vi "Impedance tube v1.0.2.vi"() -> ()   [LabVIEW 2021]
uses:
  <vilib>/Analysis/1siggen.llb/Ramp Pattern by Samples.vi
  <vilib>/express/express analysis/Spectral/Block/exnSpectralBlock spectral measurements RMS poly.vi
  <vilib>/express/express analysis/Spectral/Block/exnSpectralBlock spectral measurements RMS WFM.vi
  <vilib>/express/express analysis/Spectral/Block/exnSpectralBlock spectral measurements RMS DDT.vi
  <vilib>/Utility/file.llb/Write Delimited Spreadsheet (DBL).vi
  <vilib>/express/express arith-compare/Formula/XNode/ExpressFormulaBlockNode.xnode
  <vilib>/express/express analysis/Spectral/XNode/ExpressSpectralMeasurementsBlockNode.xnode
  <vilib>/Analysis/NI_AALPro.lvlib
  <vilib>/Analysis/NI_AALBase.lvlib
  <vilib>/measure/NI_MABase.lvlib
panel:
  out "Dout":cluster{"f0":dbl, "df":dbl, "magnitude":dbl[]}(graph)
  out "Probe":dbl[](graph)
  out "Rr":dbl[](graph)
  out "Absorption coeff":dbl[](graph)
  in  "number of samples":i32=2048
  out "MIC 2":dynamicdata(graph)
  out "MIC 2":dbl
  out "FFT1":dynamicdata(graph)
  out "MIC 1":dynamicdata(graph)
  out "MIC 1":dbl
  in  "stop (F)":bool
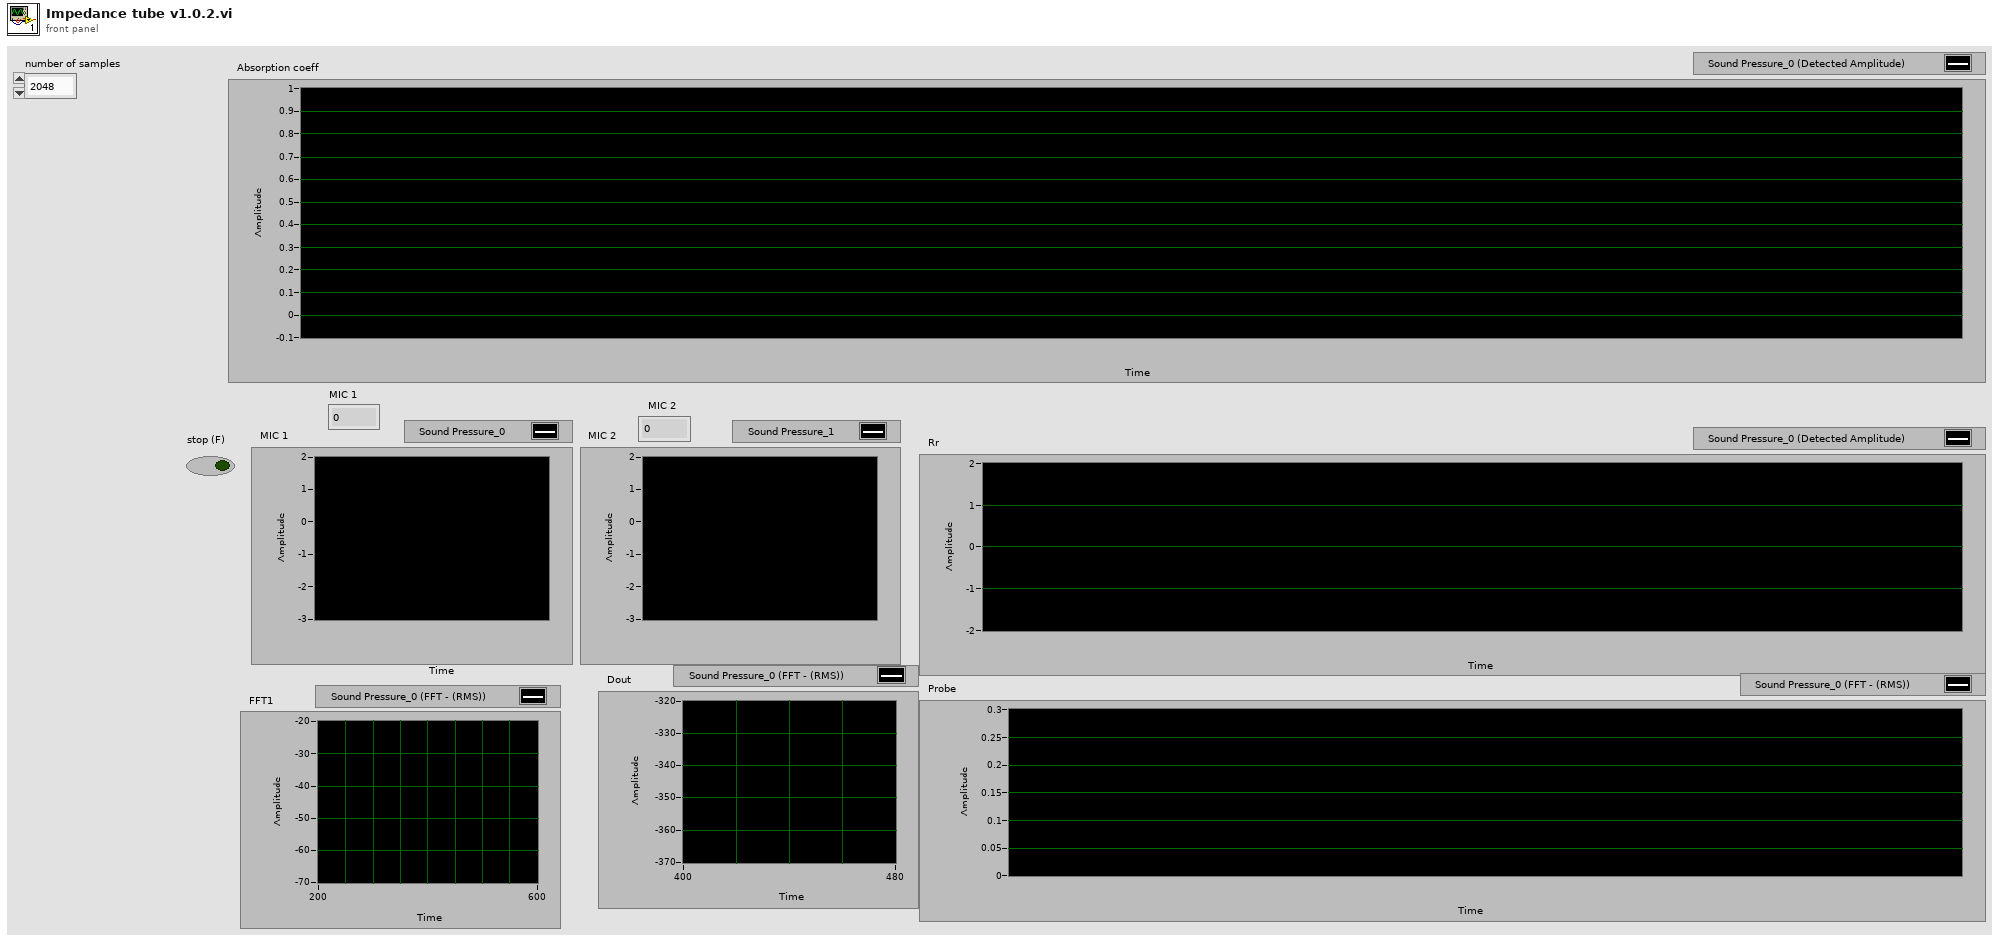
[diagram p1: front panel]
types:
  T1 = cluster{"averaging mode":u16, "weighting mode":u16, "number of averages":u32}
  T2 = cluster{"dB On (F)":bool, "unwrap phase (F)":bool, "convert to degree (F)":bool}
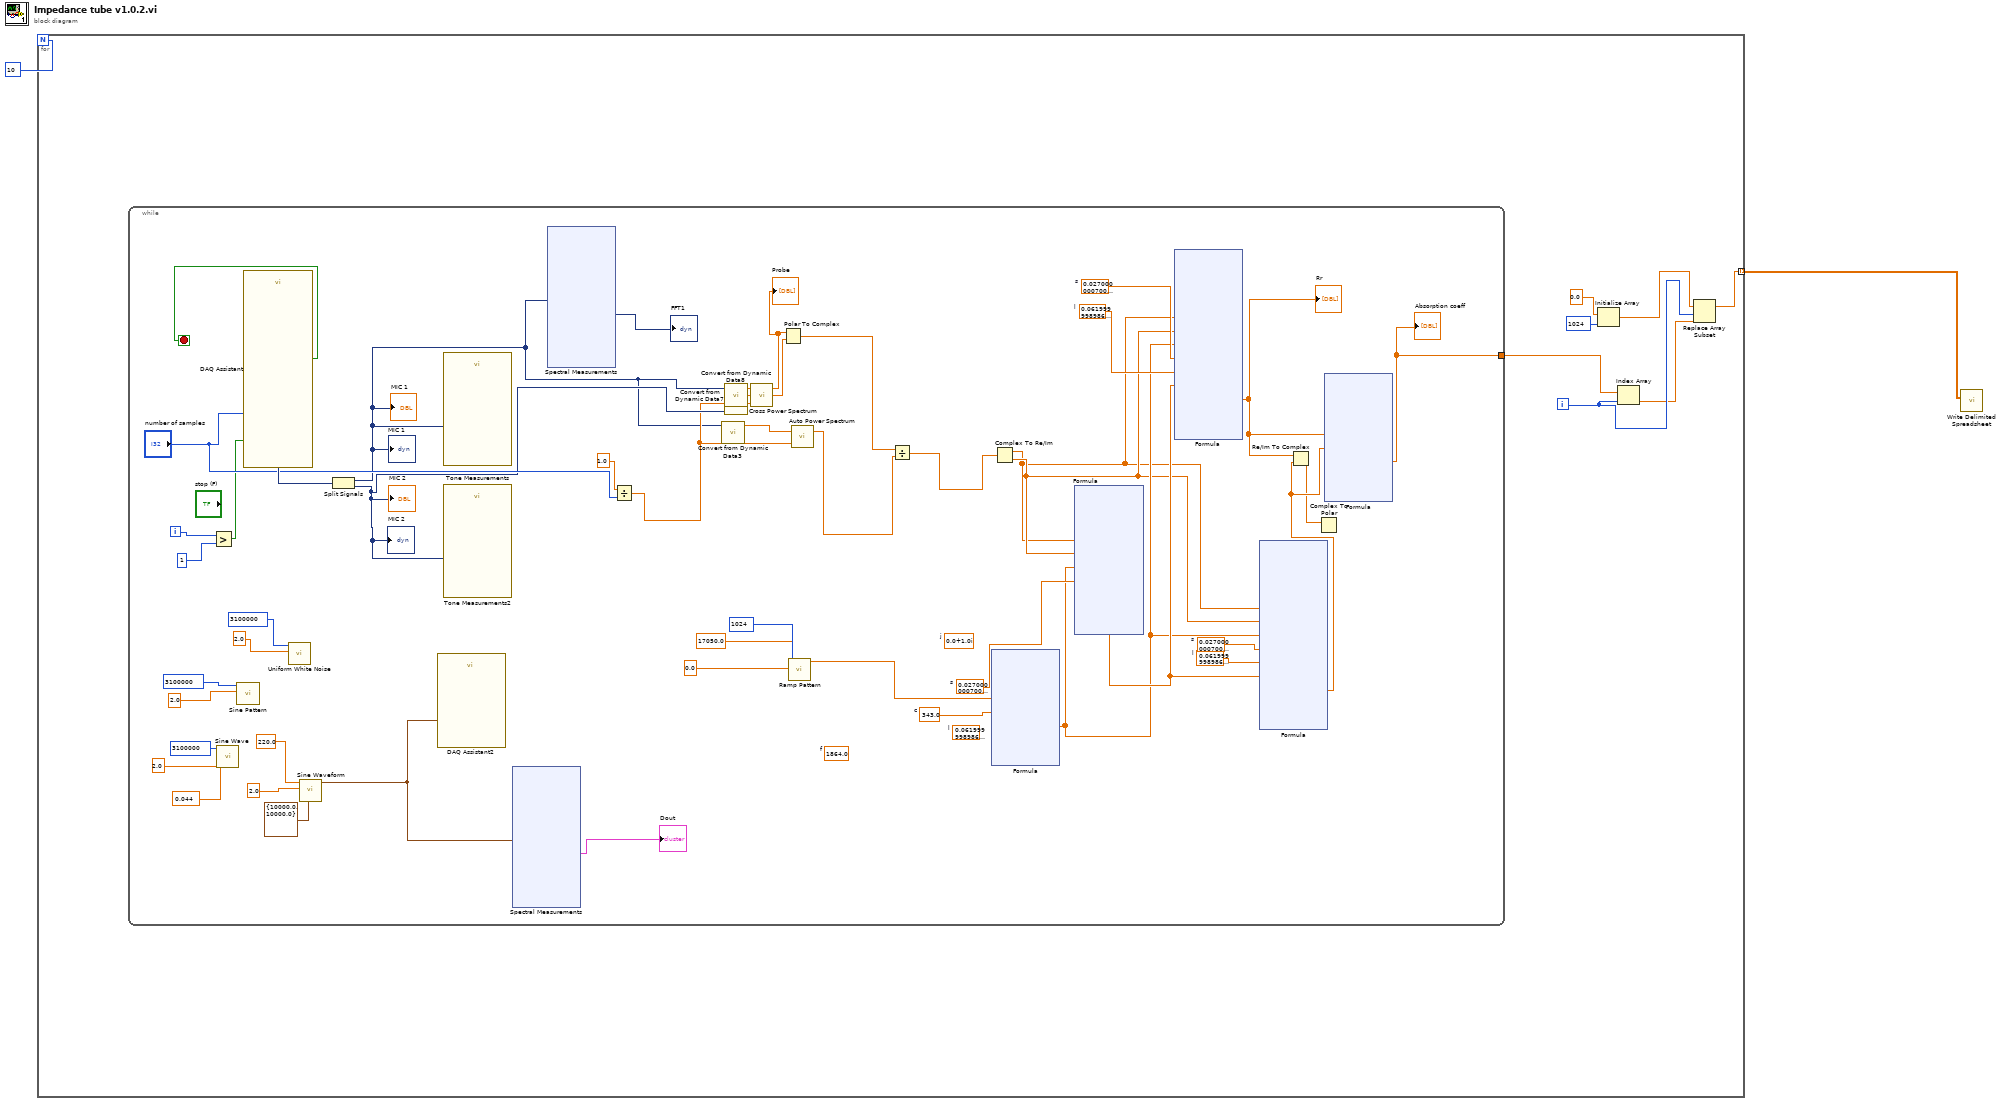
[diagram p0: block diagram]
diagram:
  n1 = for {
    N: 10 -> [_]
    tunnel: [w6] -> w1 mode=indexing
    i -> [w5]
    n2 = while {
      tunnel: [w22] -> w9
      i -> [w47]
      stop <- w23 stop-if-true
      w52 = sgl 0.062  # l
      w53 = sgl 0.027  # s
      w54 = sgl 0.062  # l
      w55 = sgl 0.027  # s
      (unwired) sgl 0.062  # l
      (unwired) sgl 1864.0  # f
      w56 = sgl 0.027  # s
      w57 = sgl 343.0  # c
      (unwired) csg 0.0+1.0i  # j
      n3 = Greater?(x=w47, y=1) -> (0:w24:bool)
      n4 = call <vilib>:"Sine Wave.vi"("samples"=3100000, "amplitude"=2.0, "frequency"=0.044) -> ()  [unwired: 2 in, 3 out]
      n5 = call <vilib>:"Sine Pattern.vi"("amplitude"=2.0, "samples"=3100000) -> ()  [unwired: 2 in, 2 out]
      n6 = call "DAQ Assistant"("number of samples"="number of samples", "stop (F)"=w24) -> ("data"=w58:dynamicdata, "stopped"=w23:bool)  [unwired: 14 in, 2 out]
      n7 = call <vilib>:"Uniform White Noise.vi"("amplitude"=2.0, "samples"=3100000) -> ()  [unwired: 8 in, 2 out]
      n8 = call <vilib>:"Sine Waveform.vi"("sampling info"=cluster{"Fs":dbl, "#s":dbl} {"Fs"=10000.0, "#s"=10000.0}, "amplitude"=2.0, "frequency"=220.0) -> ("signal out"=w11:waveform(dbl))  [unwired: 7 in, 1 out]
      n9 = Split Signals(w58) -> (w33:dynamicdata, w38:dynamicdata)  [unwired: 2 in]
      "MIC 1" <- w33
      "MIC 1" <- w33
      "MIC 2" <- w38
      "MIC 2" <- w38
      n10 = call "DAQ Assistant2"("data"=w11) -> ()  [unwired: 17 in, 2 out]
      n11 = call "Tone Measurements"("Signals"=w33) -> ()  [unwired: 8 in, 3 out]
      n12 = call "Tone Measurements2"("Signals"=w38) -> ()  [unwired: 8 in, 3 out]
      n13 = xnode "Spectral Measurements"("Signals"=w11) -> ("FFT - (RMS)"=→"Dout":cluster{"f0":dbl, "df":dbl, "magnitude":dbl[]})  [unwired: 1 in, 2 out]
      n14 = xnode "Spectral Measurements"("Signals"=w33) -> ("FFT - (RMS)"=→"FFT1":dynamicdata)  [unwired: 1 in, 2 out]
      n15 = Divide(x=1.0, y="number of samples") -> (x/y=w35:dbl)
      n16 = call "Convert from Dynamic Data3"("Dynamic Data Type"=w33) -> ("Array"=w32:dbl[])  [unwired: 3 in]
      n17 = call "Convert from Dynamic Data7"("Dynamic Data Type"=w33) -> ("Array"=w39:dbl[])  [unwired: 3 in]
      n18 = call "Convert from Dynamic Data8"("Dynamic Data Type"=w38) -> ("Array"=w37:dbl[])  [unwired: 3 in]
      n19 = call <vilib>:"Cross Power Spectrum.vi"("dt"=w35, "Signal Y (V)"=w37, "Signal X (V)"=w39) -> ("Cross Power XY Spectrum Phase (radians)"=w36:dbl[], "Cross Power XY Spectrum Mag (V^2rms)"=w34:dbl[])  [unwired: 1 out]
      "Probe" <- w34
      n20 = Polar To Complex(1:w36, 2:w34) -> (0:w31:cdb[])
      n21 = call-poly <vilib>:"Ramp Pattern.vi"("start"=0.0, "end"=17050.0, "samples"=1024) -> ("Ramp Pattern"=w25:dbl[])  [unwired: 7 in, 1 out]
      n22 = call <vilib>:"Auto Power Spectrum.vi"("dt"=w35, "Signal (V)"=w32) -> ("Power Spectrum (V^2 rms)"=w30:dbl[])  [unwired: 1 out]
      n23 = Divide(x=w31, y=w30) -> (x/y=w29:cdb[])
      n24 = xnode "Formula"("f"=w25, "c"=w57) -> ("Result"=w50:dbl[])  [unwired: 1 in, 1 out]
      n25 = Complex To Re/Im(x + iy=w29) -> (x=w44:dbl[], y=w49:dbl[])
      n26 = xnode "Formula"("Hr"=w44, "Hi"=w49, "k"=w50, "s"=w56) -> ("Result"=w51:dbl[])  [unwired: 1 in, 1 out]
      n27 = xnode "Formula"("Hr"=w44, "Hi"=w49, "k"=w50, "s"=w55, "l"=w54, "D"=w51) -> ("Result"=w41:dbl[])  [unwired: 1 in, 1 out]
      "Rr" <- w41
      n28 = xnode "Formula"("Hr"=w44, "Hi"=w49, "k"=w50, "s"=w53, "l"=w52, "D"=w51) -> ("Result"=w48:dbl[])  [unwired: 1 in, 1 out]
      n29 = Re/Im To Complex(1:w48, 2:w41) -> (0:w45:cdb[])
      n30 = Complex To Polar(r * e^(i*theta)=w45) -> ()  [unwired: 2 out]
      n31 = xnode "Formula"("Rr"=w41, "Ri"=w48) -> ("Result"=w22:dbl[])  [unwired: 1 in, 1 out]
      "Absorption coeff" <- w22
    }
    n32 = Initialize Array(0.0 ("element"), 1024 ("dimension size")) -> (w3:dbl[])
    n33 = Index Array(array=w9, index=w5) -> (element=w4:dbl)
    n34 = Replace Array Subset(array=w3, new element=w4, index=w5) -> (w6:dbl[])
  }
  n35 = call-poly <vilib>:"Write Delimited Spreadsheet.vi"("2D data"=w1) -> ()  [unwired: 13 in, 2 out]
